vi "Enable Laser.vi"(8 "error in (no error)":errorcluster, 10 "Enable Laser":bool=TRUE) -> (0 "error out":errorcluster)   [LabVIEW 2016]
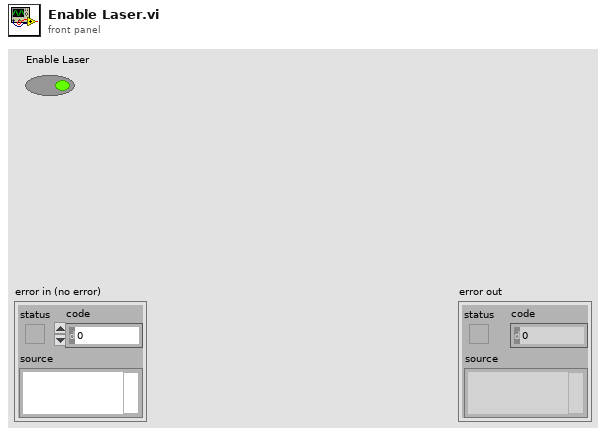
[diagram p1: front panel]
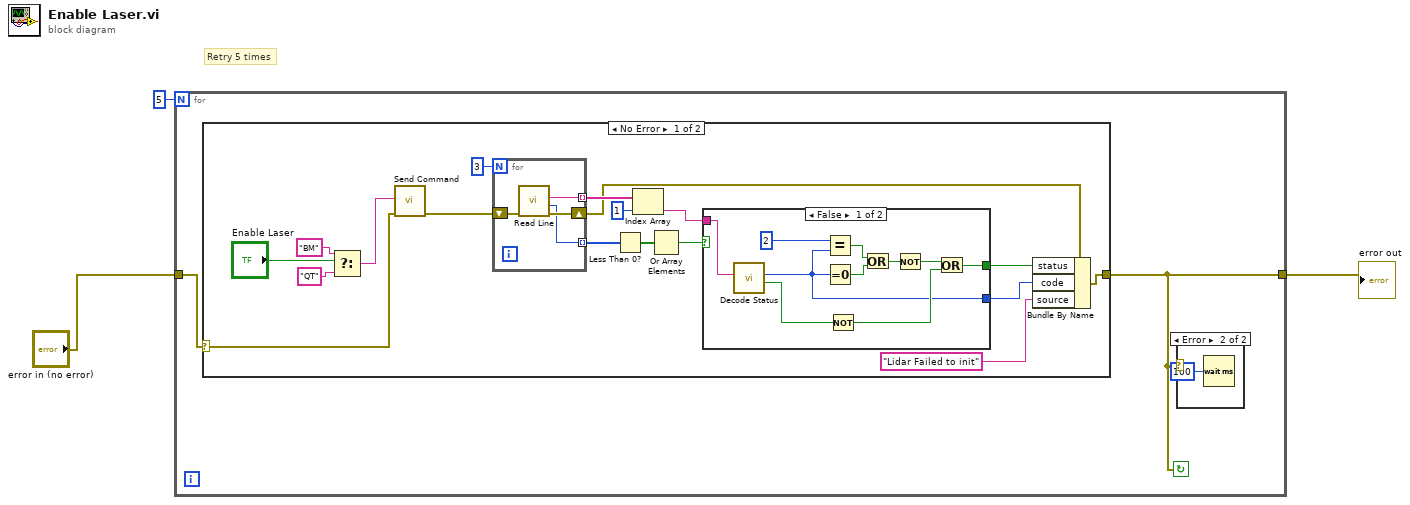
[diagram p0: block diagram]
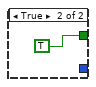
[diagram p3: hidden frame]
diagram:
  # "Retry 5 times"
  n1 = for {
    N: 5 -> [_]
    tunnel: "error in (no error)" -> [w5]
    tunnel: [w4] -> w2
    stop <- w4 continue-if-true
    n2 = case shown="No Error" w5 {
      selector: w5 -> [w10 w40]
      tunnel: [w14 w40] -> w4
      frame No Error {
        n3 = Select(t="BM", s="Enable Laser", f="QT") -> (s? t:f=w11:string)
        n4 = call "Send Command.vi"("error in (no error)"=w10, "Command"=w11) -> ("error out"=w9:errorcluster)  [unwired: 9 in]
        n5 = for {
          N: 3 -> [_]
          tunnel: [w37] -> w20 mode=indexing
          tunnel: [w36] -> w23 mode=indexing
          shift-right: [w38] -> w8
          shift-left: w9 -> [w39]
          n6 = call "Read Line.vi"("error in (no error)"=w39) -> ("error out"=w38:errorcluster, "Line length"=w36:i32, "Line"=w37:string)  [unwired: 8 in]
        }
        n7 = Less Than 0?(x=w23) -> (x < 0?=w22:bool[])
        n8 = Index Array(array=w20, index=1) -> (element=w18:string)
        n9 = Or Array Elements(Boolean array=w22) -> (logical OR=w21:bool)
        n10 = case shown="False" w21 {
          tunnel: w18 -> [w27 _]
          tunnel: [w33 TRUE] -> w13
          tunnel: [w26 _] -> w12
          frame False {
            n11 = call "Decode Status.vi"("Status Line"=w27) -> ("Checksum OK"=w25:bool, "Output"=w26:i32)  [unwired: 8 in, 1 out]
            n12 = Equal?(x=2, y=w26) -> (x = y?=w31:bool)
            n13 = Equal To 0?(x=w26) -> (x = 0?=w32:bool)
            n14 = Not(x=w25) -> (.not. x?=w34:bool)
            n15 = Or(x=w31, y=w32) -> (x .or. y?=w29:bool)
            n16 = Not(x=w29) -> (.not. x?=w28:bool)
            n17 = Or(x=w28, y=w34) -> (x .or. y?=w33:bool)
          }
          frame True {
          }
        }
        n18 = Bundle By Name(cluster=w8, "status"=w13, "code"=w12, "source"="Lidar Failed to init") -> (w14:errorcluster)
      }
      frame Error {
      }
    }
    n19 = case shown="Error" w4 {
      frame No Error {
      }
      frame Error {
        n20 = Wait (ms)(milliseconds to wait=u32 100) -> ()  [unwired: 1 out]
      }
    }
  }
  "error out" <- w2
